vi "全局 多参数.vi"() -> ()   [LabVIEW 2016]
panel:
  in  "多参数":string[][](array[string])
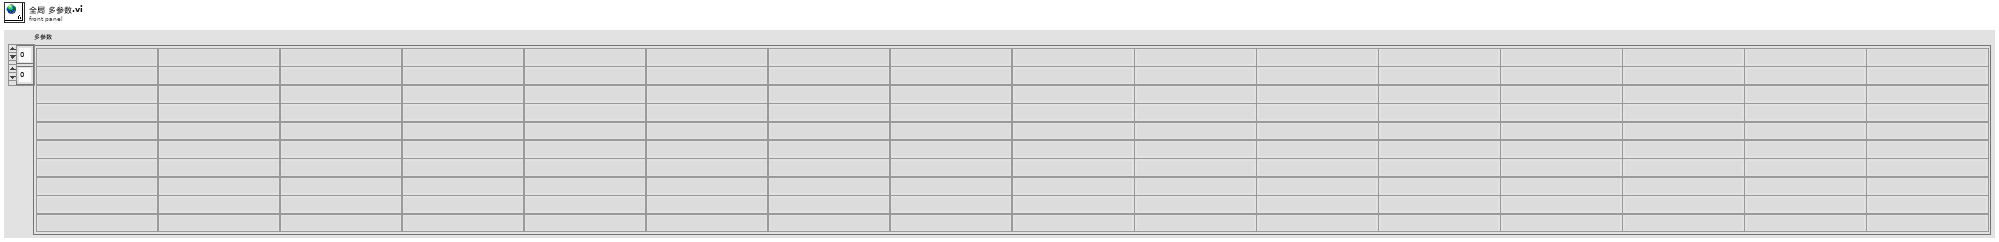
[diagram p1: front panel]
diagram:
